vi "HEWH Calibration File Check.vi"(8 "error in (no error)":errorcluster, 11 "Calibration Path":path) -> (0 "error out":errorcluster={"status"=TRUE, "code"=-1073807346, "source"="VISA Read in Gather Test Data.vi"}, 1 "Calibration Path":path, 2 "Calibration File Array":dbl[][](array[numeric]), 3 "Complete File?":bool)   [LabVIEW 2019]
uses:
  <vilib>/Utility/file.llb/Read From Spreadsheet File (string).vi
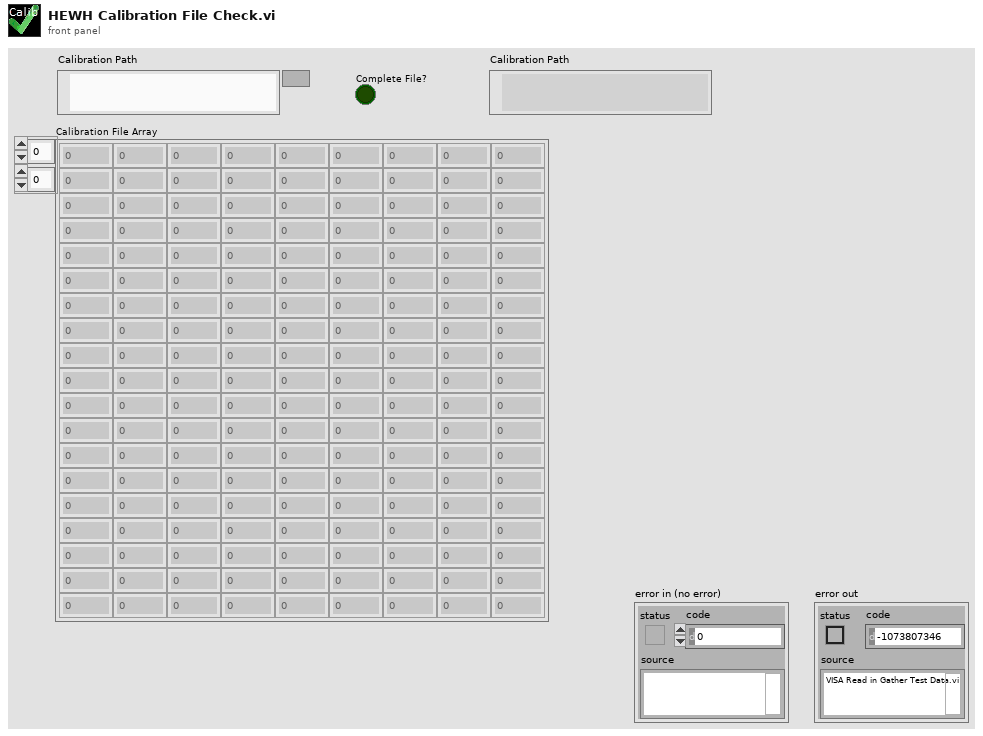
[diagram p1: front panel]
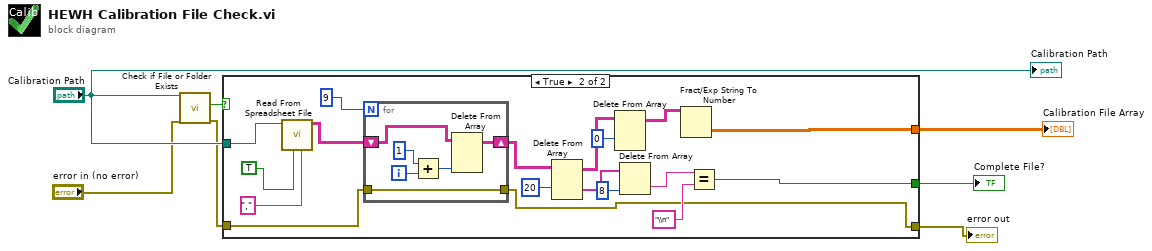
[diagram p0: block diagram]
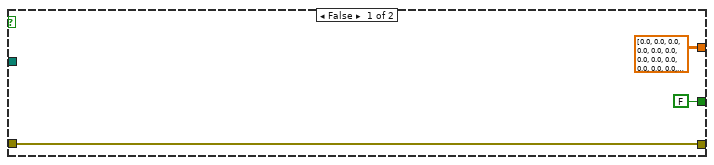
[diagram p2: hidden frame]
diagram:
  n1 = call <vilib>:"Check if File or Folder Exists.vi"("error in (no error)"="error in (no error)", "path"="Calibration Path") -> ("error out"=w2:errorcluster, "file or folder exists?"=w6:bool)  [unwired: 7 in, 1 out]
  n2 = case shown="True" w6 {
    tunnel: "Calibration Path" -> [_ w28]
    tunnel: [dbl[][] [[0.0, 0.0, 0.0, 0.0, 0.0, 0.0, 0.0, 0.0, 0.0], [0.0, 0.0, 0.0, 0.0, 0.0, 0.0, 0.0, 0.0, 0.0], [0.0, 0.0, 0.0, 0.0, 0.0, 0.0, 0.0, 0.0, 0.0], [0.0, 0.0, 0.0, 0.0, 0.0, 0.0, 0.0, 0.0, 0.0], [0.0, 0.0, 0.0, 0.0, 0.0, 0.0, 0.0, 0.0, 0.0], [0.0, 0.0, 0.0, 0.0, 0.0, 0.0, 0.0, 0.0, 0.0], [0.0, 0.0, 0.0, 0.0, 0.0, 0.0, 0.0, 0.0, 0.0], [0.0, 0.0, 0.0, 0.0, 0.0, 0.0, 0.0, 0.0, 0.0], [0.0, 0.0, 0.0, 0.0, 0.0, 0.0, 0.0, 0.0, 0.0], [0.0, 0.0, 0.0, 0.0, 0.0, 0.0, 0.0, 0.0, 0.0], [0.0, 0.0, 0.0, 0.0, 0.0, 0.0, 0.0, 0.0, 0.0], [0.0, 0.0, 0.0, 0.0, 0.0, 0.0, 0.0, 0.0, 0.0], [0.0, 0.0, 0.0, 0.0, 0.0, 0.0, 0.0, 0.0, 0.0], [0.0, 0.0, 0.0, 0.0, 0.0, 0.0, 0.0, 0.0, 0.0], [0.0, 0.0, 0.0, 0.0, 0.0, 0.0, 0.0, 0.0, 0.0], [0.0, 0.0, 0.0, 0.0, 0.0, 0.0, 0.0, 0.0, 0.0], [0.0, 0.0, 0.0, 0.0, 0.0, 0.0, 0.0, 0.0, 0.0], [0.0, 0.0, 0.0, 0.0, 0.0, 0.0, 0.0, 0.0, 0.0], [0.0, 0.0, 0.0, 0.0, 0.0, 0.0, 0.0, 0.0, 0.0]] w14] -> w4
    tunnel: [FALSE w13] -> w5
    tunnel: w2 -> [w8 w12]
    tunnel: [w8 w11] -> w1
    frame False {
    }
    frame True {
      n3 = call-poly <vilib>:"Read From Spreadsheet File.vi"("delimiter (\\t)"="," ("delimiter (\\t)"), "transpose (no:F)"=TRUE, "file path (dialog if empty)"=w28) -> ("all rows"=w24:string[][])  [unwired: 4 in, 4 out]
      n4 = for {
        N: 9 -> [_]
        shift-right: [w33] -> w23
        shift-left: w24 -> [w34]
        tunnel: w12 -> [w29]
        tunnel: [w29] -> w11
        i -> [w32]
        n5 = Add(x=1 ("disabled index (col)"), y=w32) -> (x+y=w30:i32)
        n6 = Delete From Array(array=w34, index (col)=w30) -> (array with subset deleted=w33:string[][])  [unwired: 2 in, 1 out]
      }
      n7 = Delete From Array(array=w23, index (row)=20) -> (deleted portion=w21:string[], array with subset deleted=w17:string[][])  [unwired: 2 in]
      n8 = Delete From Array(array=w17, index (row)=0) -> (array with subset deleted=w15:string[][])  [unwired: 2 in, 1 out]
      n9 = Delete From Array(array=w21, index=8) -> (deleted portion=w19:string)  [unwired: 1 in, 1 out]
      n10 = Fract/Exp String To Number(string=w15) -> (number=w14:dbl[][])  [unwired: 3 in, 1 out]
      n11 = Equal?(x=w19, y="\\n") -> (x = y?=w13:bool)
    }
  }
  "Calibration File Array" <- w4
  "Complete File?" <- w5
  "error out" <- w1
  "Calibration Path" <- "Calibration Path"
